vi "GrabAllDataSynthFoc.vi"(4 "All files":string[](array[string]), 5 "error in":errorcluster, 6 "lines per plane mod":i32, 7 "Synth Foc?":bool, 8 "save?":bool=TRUE, 9 "Xmit Ring":i16, 10 "Start Record":i32, 11 "Reverse ?":bool) -> (12 "Gain Array":T1(array[cluster]), 14 "SA Data Out":refnum<data-value>, 15 "Raw data out":i16[][][](array[numeric]), 19 "error out":errorcluster)   [LabVIEW 2022 SP3]
uses:
  ScanningControl/Motion Controllers/-MotionRoutines/MotionGlobals.vi
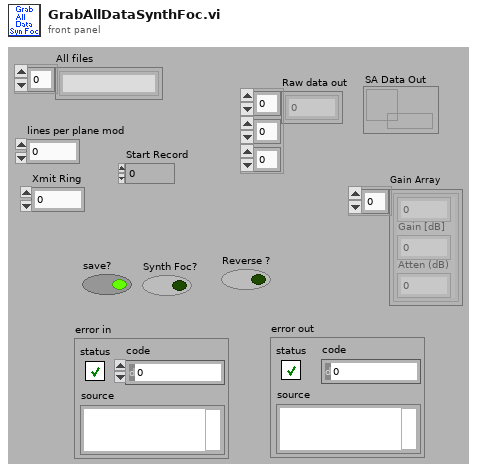
[diagram p1: front panel]
types:
  T1 = cluster{sgl, "Gain [dB]  ":sgl, "Atten (dB)":sgl}[]
  T2 = cluster{sgl, "Gain [dB]  ":sgl, "Atten (dB)":sgl}[][]
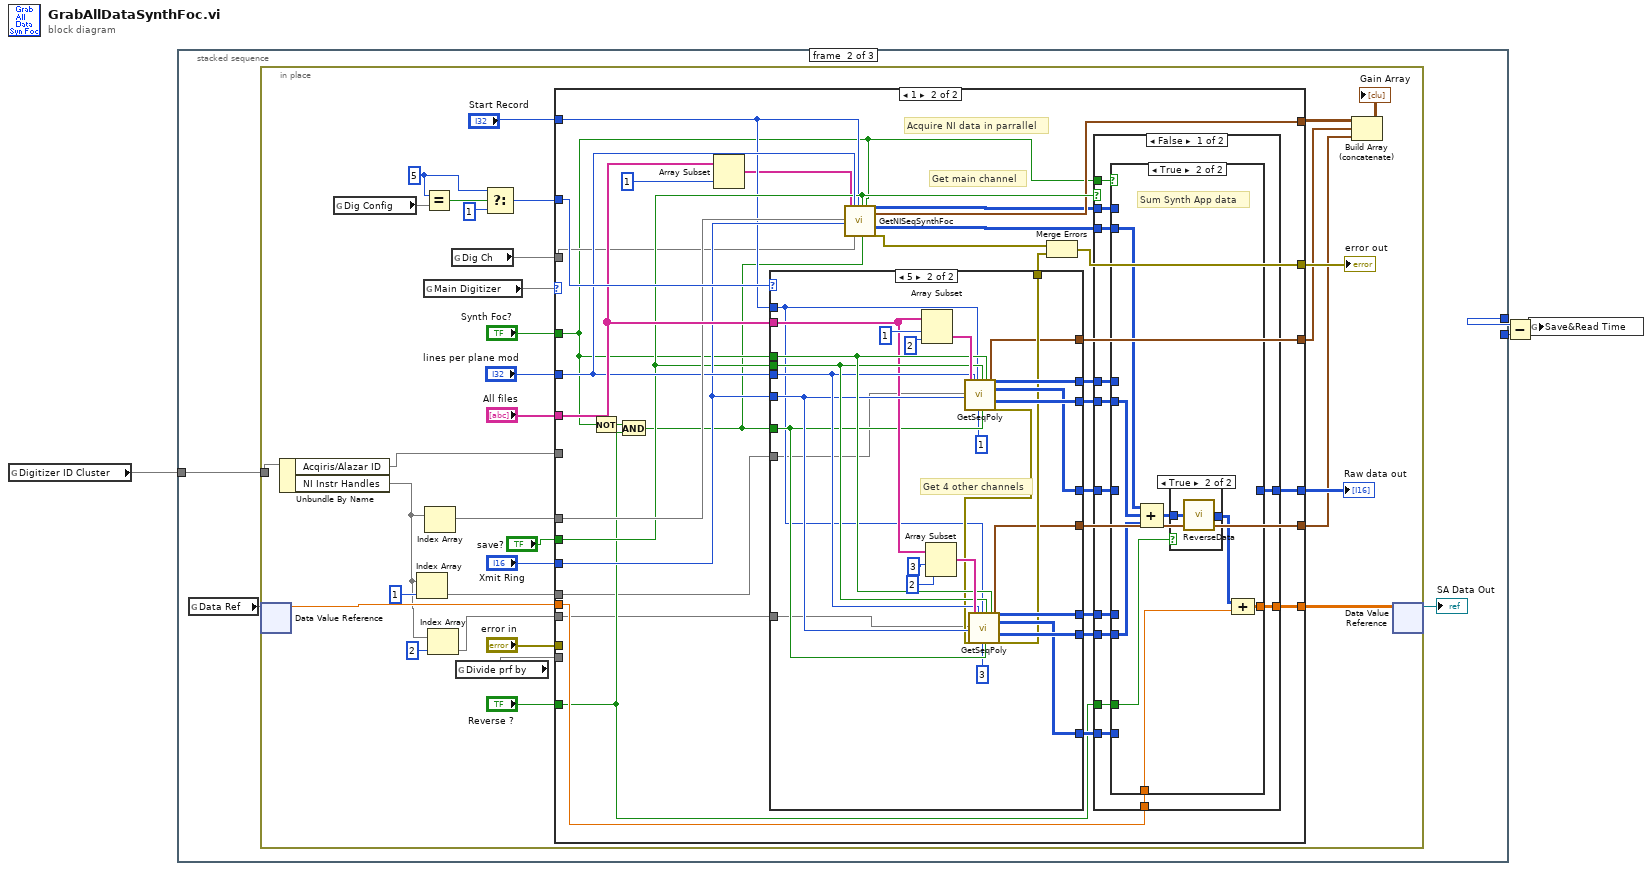
[diagram p0: block diagram]
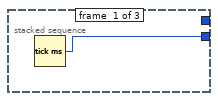
[diagram p2: hidden frame]
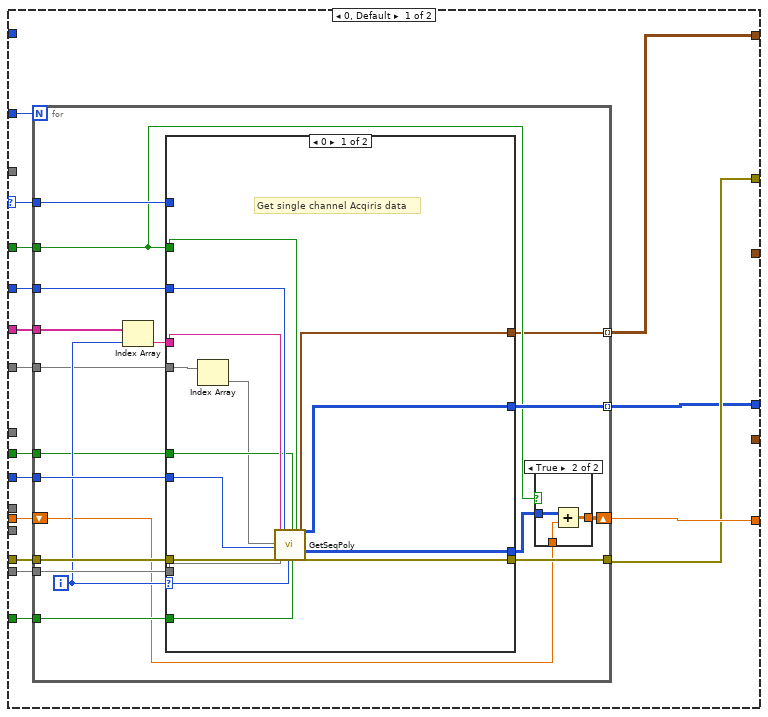
[diagram p3: hidden frame]
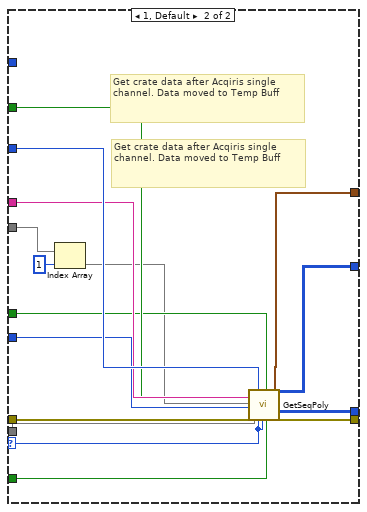
[diagram p5: hidden frame]
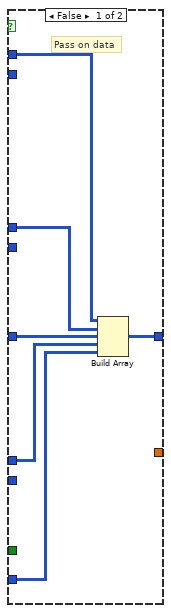
[diagram p6: hidden frame]
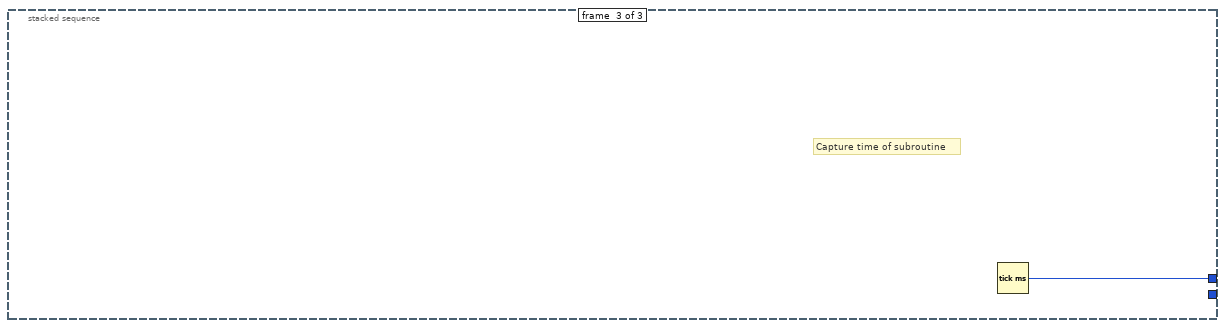
[diagram p10: hidden frame]
diagram:
  n1 = global read "MotionGlobals.vi" "Digitizer ID Cluster"() -> (w1)
  n2 = stacked-sequence {
    tunnel: [w5 _ _] -> w3
    tunnel: [_ _ w200] -> w2
    tunnel: w1 -> [_ w6 _]
    frame #0 {
      n3 = Tick Count (ms)() -> (millisecond timer value=w5:u32)
    }
    frame #1 {
      n4 = global read "MotionGlobals.vi" "Data Ref"() -> (w8)
      n5 = in-place {
        in-place-border: w6 -> [w10]
        w40 = 5
        n6 = in-place-dvr #1(w8) -> (w19:dbl)  [unwired: 1 out]
        n7 = Unbundle By Name(w10) -> ("Acqiris/Alazar ID"=w9, "NI Instr Handles"=w11)
        n8 = global read "MotionGlobals.vi" "Dig Config"() -> (w29)
        n9 = Index Array(array=w11, index=1) -> (element=w13)
        n10 = Equal?(x=w40, y=w29) -> (x = y?=w39:bool)
        n11 = global read "MotionGlobals.vi" "Main Digitizer"() -> (w26)
        n12 = Index Array(array=w11) -> (element=w16)  [unwired: 1 in]
        n13 = Index Array(array=w11, index=2) -> (element=w12)
        n14 = global read "MotionGlobals.vi" "Dig Ch"() -> (w24)
        n15 = global read "MotionGlobals.vi" "Divide prf by"() -> (w28)
        n16 = Select(t=w40, s=w39, f=1) -> (s? t:f=w37:i32)
        n17 = case shown="1" w26 {
          selector: w26 -> [w43 _]
          tunnel: "All files" -> [w56 w141]
          tunnel: w37 -> [w55 w142]
          tunnel: [w54 w136] -> w18
          tunnel: "Xmit Ring" -> [w53 w138]
          tunnel: w19 -> [w52 w134]
          tunnel: "Synth Foc?" -> [w51 w115]
          tunnel: "Reverse ?" -> [w50 w112]
          tunnel: [w49 w133] -> w32
          tunnel: "lines per plane mod" -> [w48 w139]
          tunnel: "error in" -> [w47 _]
          tunnel: w16 -> [_ w140]
          tunnel: w28 -> [w46 _]
          tunnel: [w45 w135] -> w27
          tunnel: "save?" -> [w44 w137]
          tunnel: "Start Record" -> [_ w132]
          tunnel: w24 -> [_ w131]
          tunnel: [w42 w130] -> w23
          tunnel: [_ w129] -> w22
          tunnel: [_ w128] -> w21
          tunnel: w13 -> [_ w111]
          tunnel: w12 -> [_ w110]
          tunnel: w9 -> [w41 _]
          frame 0, Default {
            n18 = for {
              N: w55 -> [_]
              tunnel: w46 -> [w74]
              tunnel: w47 -> [w73]
              tunnel: w48 -> [w72]
              tunnel: [w71] -> w49
              tunnel: w50 -> [w70]
              tunnel: w51 -> [w62]
              tunnel: w53 -> [w69]
              shift-right: [w60] -> w54
              shift-left: w52 -> [w59]
              tunnel: w56 -> [w66]
              tunnel: w43 -> [w65]
              tunnel: [w64] -> w45 mode=indexing
              tunnel: w44 -> [w63]
              tunnel: [w58] -> w42 mode=indexing
              tunnel: w41 -> [w57]
              i -> [w67]
              n19 = Index Array(array=w66, index=w67) -> (element=w68:string)
              n20 = case shown="0" w67 {
                selector: w67 -> [w84 w101]
                tunnel: w74 -> [w93 w102]
                tunnel: w73 -> [w92 w109]
                tunnel: w72 -> [w91 w108]
                tunnel: [w86 w105] -> w71
                tunnel: w70 -> [w90 w107]
                tunnel: w62 -> [w89 w104]
                tunnel: w69 -> [w85 w103]
                tunnel: [w87 w98] -> w61
                tunnel: w68 -> [w88 w106]
                tunnel: w65 -> [_ _]
                tunnel: [w83 w100] -> w64
                tunnel: w63 -> [w82 w99]
                tunnel: [w81 w97] -> w58
                tunnel: w57 -> [w80 w95]
                frame 0 {
                  # "Get single channel Acqiris data"
                  n21 = Index Array(array=w80) -> (element=w79)  [unwired: 1 in]
                  n22 = call-poly "GetSeqPoly.vi"("NI Card"=w79, 4:w85, "errorin"=w92, "File Array"=w88, "Ann Array Params"=w93, "lines per plane"=w91, "Rcv Ring"=w84, "save?"=w82, "Reverse?"=w90, 16:w89) -> ("Gain Array"=w81:T1, "Array"=w83:i8[][], "Synth App Out"=w87:i16[][], "error out"=w86:errorcluster)  [unwired: 4 in, 10 out]
                }
                frame 1, Default {
                  # "Get crate data after Acqiris single channel. Data moved to Temp Buff"
                  # "Get crate data after Acqiris single channel. Data moved to Temp Buff"
                  n23 = Index Array(array=w95, index=1) -> (element=w94)
                  n24 = call-poly "GetSeqPoly.vi"("NI Card"=w94, 4:w103, "errorin"=w109, "File Array"=w106, "Ann Array Params"=w102, "lines per plane"=w108, "Channel (0)"=w101, "Rcv Ring"=w101, "save?"=w99, "Reverse?"=w107, 16:w104) -> ("Gain Array"=w97:T1, "Array"=w100:i8[][], "Synth App Out"=w98:i16[][], "error out"=w105:errorcluster)  [unwired: 3 in, 10 out]
                }
              }
              n25 = case shown="True" w62 {
                tunnel: w61 -> [w75 w77]
                tunnel: [w75 w78] -> w60
                tunnel: w59 -> [_ w76]
                frame False {
                }
                frame True {
                  n26 = Add(x=w77, y=w76) -> (x+y=w78:dbl[][])
                }
              }
            }
          }
          frame 1 {
            # "Acquire NI data in parrallel"
            # "Get main channel"
            n27 = Not(x=w115) -> (.not. x?=w113:bool)
            n28 = And(x=w113, y=w112) -> (x .and. y?=w114:bool)
            n29 = Array Subset(array=w141, length=1) -> (w127:string[])  [unwired: 1 in]
            n30 = case shown="5" w142 {
              tunnel: w141 -> [_ w191]
              tunnel: w114 -> [_ w182]
              tunnel: w138 -> [_ w192]
              tunnel: w115 -> [_ w195]
              tunnel: w137 -> [_ w194]
              tunnel: w139 -> [_ w193]
              tunnel: [_ w190] -> w123
              tunnel: [_ w189] -> w125
              tunnel: [_ w184] -> w122
              tunnel: [_ w188] -> w121
              tunnel: [_ w187] -> w124
              tunnel: [_ w183] -> w120
              tunnel: [_ w181] -> w117
              tunnel: w132 -> [_ w175]
              tunnel: [_ w178] -> w129
              tunnel: [_ w177] -> w128
              tunnel: w111 -> [_ w174]
              tunnel: w110 -> [_ w173]
              frame 0, Default {
              }
              frame 5 {
                # "Get 4 other channels"
                n31 = Array Subset(array=w191, index=1, length=2) -> (w198:string[])
                n32 = Array Subset(array=w191, index=3, length=2) -> (w196:string[])
                n33 = call-poly "GetSeqPoly.vi"("NI Card"=w174, 4:w192, "File Array"=w198, "lines per plane"=w193, "Start Record"=w175, "Rcv Ring"=1, "save?"=w194, "Reverse?"=w182, 16:w195) -> ("Gain Array"=w178:T1, "Array"=w190:i8[][], "Array 2"=w184:i8[][], "Synth App Out"=w189:i16[][], "error out"=w176:errorcluster)  [unwired: 5 in, 9 out]
                n34 = call-poly "GetSeqPoly.vi"("NI Card"=w173, 4:w192, "errorin"=w176, "File Array"=w196, "lines per plane"=w193, "Start Record"=w175, "Rcv Ring"=3, "save?"=w194, "Reverse?"=w182, 16:w195) -> ("Gain Array"=w177:T1, "Array"=w188:i8[][], "Array 2"=w183:i8[][], "Synth App Out"=w187:i16[][], "error out"=w181:errorcluster)  [unwired: 4 in, 9 out]
              }
            }
            n35 = call "GetNISeqSynthFoc.vi"("NI Card"=w140, 4:w138, "File Array"=w127, "lines per plane"=w139, "Channel (0)"=w131, "Start Record"=w132, "save?"=w137, "Reverse?"=w114, 16:w115) -> ("Gain Array"=w130:T1, "Array"=w126:i8[][], "Synth App Out"=w116:i16[][], "error out"=w118:errorcluster)  [unwired: 7 in, 8 out]
            n36 = Merge Errors(w118, w117) -> (w133:errorcluster)
            n37 = case shown="False" w137 {
              tunnel: w126 -> [w150 _]
              tunnel: w116 -> [w154 _]
              tunnel: w115 -> [w155 _]
              tunnel: w125 -> [w153 _]
              tunnel: w124 -> [w152 _]
              tunnel: [w151 _] -> w136
              tunnel: w123 -> [w149 _]
              tunnel: w122 -> [w148 _]
              tunnel: w121 -> [w147 _]
              tunnel: w120 -> [w146 _]
              tunnel: [w145 _] -> w135
              tunnel: w134 -> [w144 _]
              tunnel: w112 -> [w143 _]
              frame False {
                n38 = case shown="True" w155 {
                  tunnel: w154 -> [_ w169]
                  tunnel: w153 -> [_ w168]
                  tunnel: w152 -> [_ w167]
                  tunnel: [_ w162] -> w151
                  tunnel: w150 -> [w161 _]
                  tunnel: w149 -> [w160 _]
                  tunnel: w148 -> [w159 _]
                  tunnel: w147 -> [w158 _]
                  tunnel: w146 -> [w157 _]
                  tunnel: [w156 _] -> w145
                  tunnel: w144 -> [_ w163]
                  tunnel: w143 -> [_ w165]
                  frame False {
                    # "Pass on data"
                    n39 = Build Array(w161, w160, w159, w158, w157) -> (w156:i8[][][])
                  }
                  frame True {
                    # "Sum Synth App data"
                    n40 = Compound Arithmetic op=ADD(w169, w168, w167) -> (w166:i16[][])
                    n41 = case shown="True" w165 {
                      tunnel: w166 -> [w170 w172]
                      tunnel: [w170 w171] -> w164
                      frame False {
                      }
                      frame True {
                        n42 = call "ReverseData.vi"("Array in"=w172) -> ("Array out"=w171:i16[][])
                      }
                    }
                    n43 = Compound Arithmetic op=unknown(w164, w163) -> (w162:dbl[][])
                  }
                }
              }
              frame True {
              }
            }
          }
        }
        "error out" <- w32
        "Raw data out" <- w27
        n44 = Build Array (concatenate)(w23, w22, w21) -> (→"Gain Array":T2)
        n45 = in-place-dvr #1(w18) -> (→"SA Data Out":refnum<data-value>)  [unwired: 1 out]
      }
    }
    frame #2 {
      # "Capture time of subroutine"
      n46 = Tick Count (ms)() -> (millisecond timer value=w200:u32)
    }
  }
  n47 = Subtract(x=w2, y=w3) -> (x-y=w4:u32)
  n48 = global write "MotionGlobals.vi" "Save&Read Time"(w4) -> ()
